vi "Core.vi"(8 "error in (no error)":errorcluster, 11 "Serial in":refnum<class "Serial.lvclass">) -> (0 "error out":errorcluster, 3 "Serial out":refnum<class "Serial.lvclass">)   [LabVIEW 2021, in "Serial.lvclass"]
uses:
  Serial.lvclass
  D:/my_projects/projects/Algorithms/Labview/21/Modbus_v121c/Network Protocol/MB/Modbus Master CR.lvclass
  MB/ctl/MB_TCP_State.ctl
  MB/Modbus Master CR.lvclass/Modbus Master CR.ctl
  MB/Status/Run/Write Run.vi
  MB/Status/write/Write write.vi
  Data Model/Device Data Model.lvclass
  MB/Modbus Master CR.lvclass
panel:
  out "MB_TCP_State":T1=enum."requests"
  in  "write enable":bool=TRUE
  in  "stop":bool
  out "stopped":bool
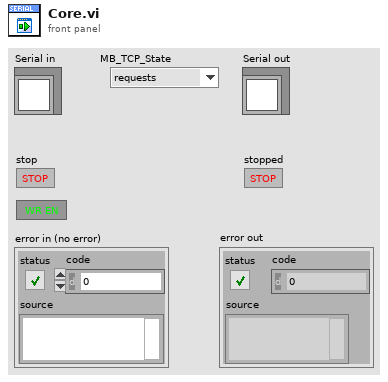
[diagram p1: front panel]
types:
  T1 = typedef "Modbus Master CR.lvclass/MB_TCP_State.ctl" = enum8{"initialization", "redefine", "standby", "ping", "connect", "wait to reconnect", "wait to reset timeout", "configure", "requests", "close connection", "stop"}
  T2 = typedef "Modbus Master CR.lvclass/MB timeouts.ctl" = cluster{"reconn_timeout":i32, "N attempt max":i32, "t_reset_TTL":i32, "period":i32}
  T3 = typedef "Modbus Master CR.lvclass/MB state.ctl" = cluster{"state":T1, "enable":bool, "Run":bool, "write enable":bool, "Write":bool, "connect":bool, "errors":i32}
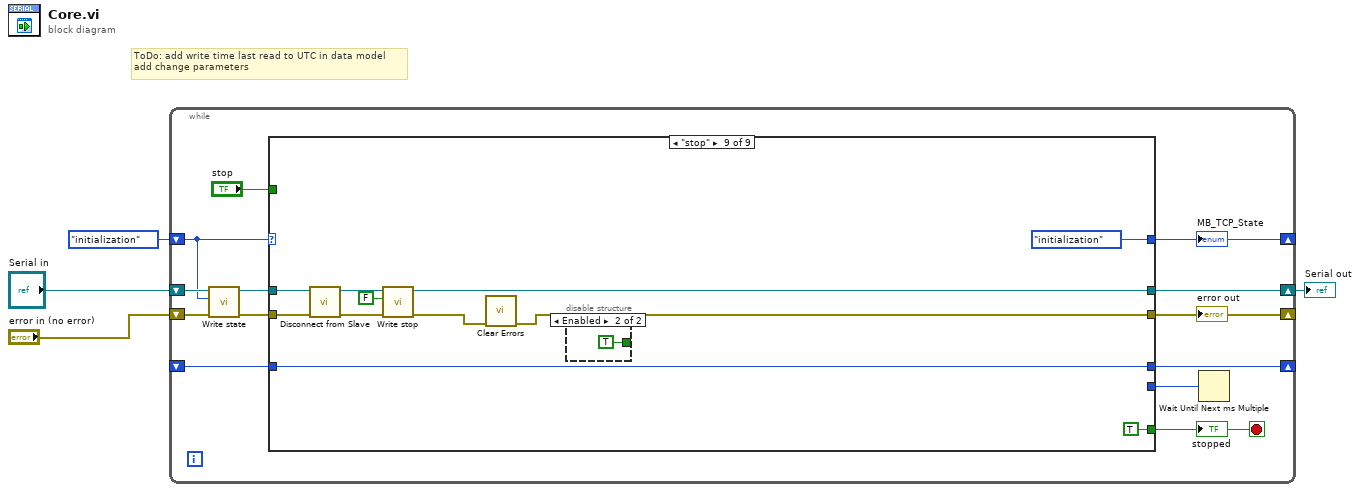
[diagram p0: block diagram]
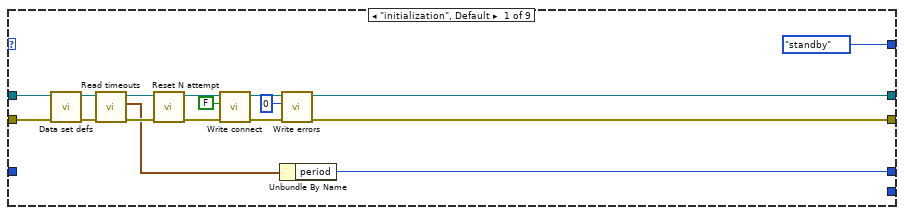
[diagram p2: hidden frame]
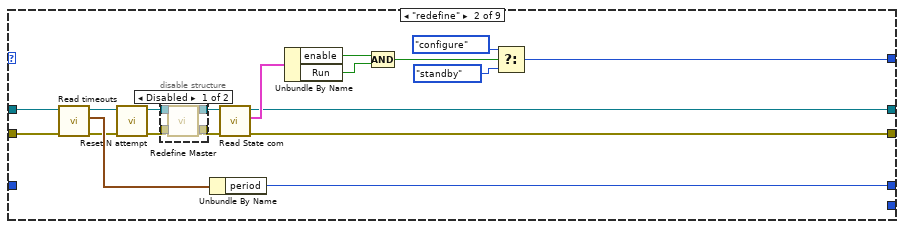
[diagram p3: hidden frame]
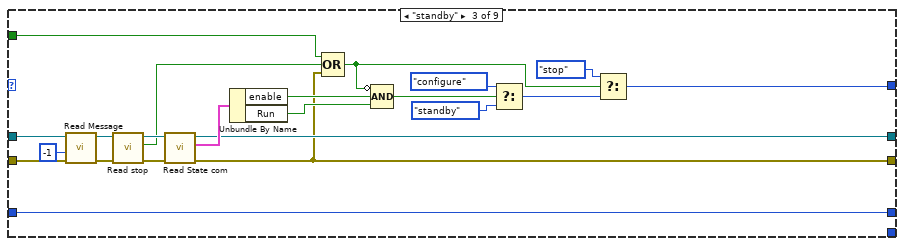
[diagram p5: hidden frame]
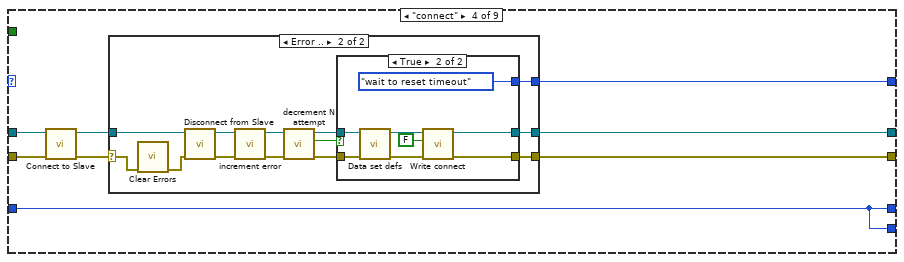
[diagram p6: hidden frame]
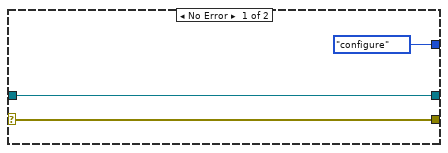
[diagram p7: hidden frame]
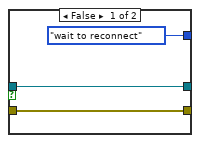
[diagram p8: hidden frame]
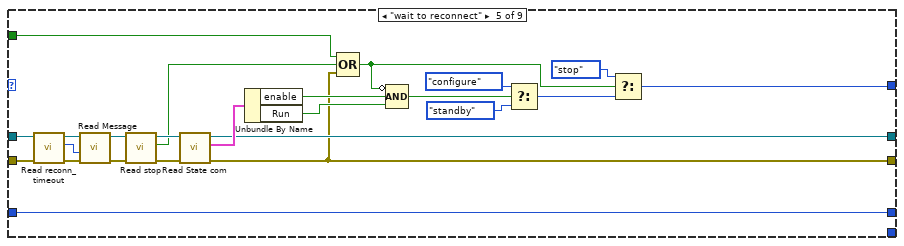
[diagram p9: hidden frame]
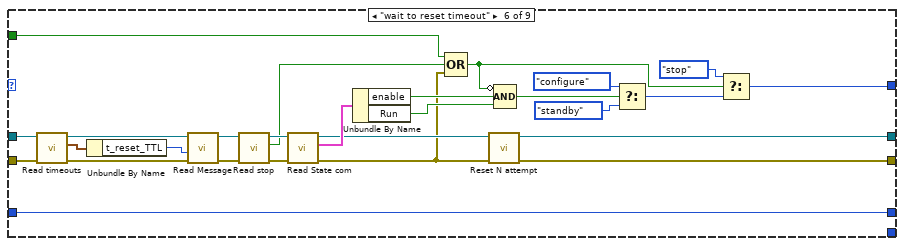
[diagram p10: hidden frame]
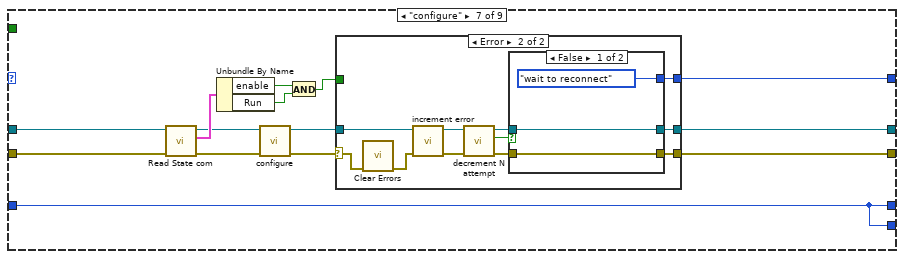
[diagram p11: hidden frame]
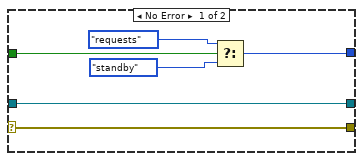
[diagram p12: hidden frame]
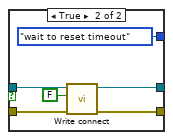
[diagram p13: hidden frame]
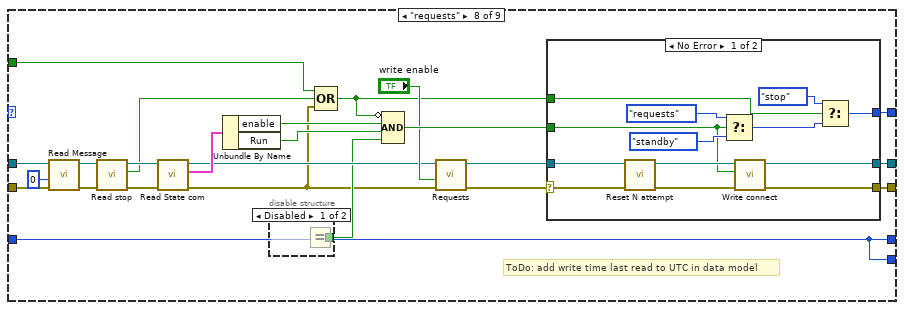
[diagram p14: hidden frame]
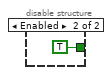
[diagram p15: hidden frame]
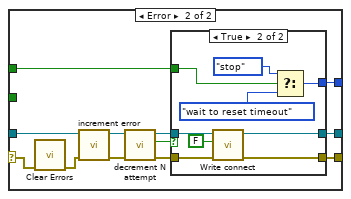
[diagram p16: hidden frame]
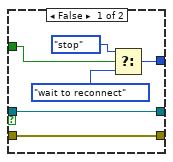
[diagram p17: hidden frame]
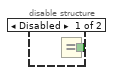
[diagram p18: hidden frame]
diagram:
  # "ToDo: add write time last read to UTC in data model\nadd change parameters"
  n1 = while {
    shift-right: [w10] -> w4
    shift-left: "Serial in" -> [w9]
    shift-right: [w11] -> _
    shift-left: "error in (no error)" -> [w7]
    shift-right: [w15] -> _
    shift-left: _ -> [w16]
    shift-right: [w12] -> _
    shift-left: MB_TCP_State."initialization" ("state") -> [w5]
    stop <- w17 stop-if-true
    n2 = call "Write state.vi"("error in (no error)"=w7, "state"=w5, "MB in"=w9) -> ("error out"=w6:errorcluster, "MB out"=w8:refnum<class "Serial.lvclass">)  [unwired: 7 in]
    n3 = case shown="\"stop\"" w5 {
      tunnel: "stop" -> [_ _ w77 _ w125 w151 _ w220 _]
      tunnel: [_ _ _ _ _ _ _ _ TRUE] -> w17
      tunnel: w8 -> [w31 w50 w67 w85 w139 w166 w174 w223 w283]
      tunnel: [w20 w36 w69 w89 w123 w143 w181 w230 w276] -> w10
      tunnel: w6 -> [w32 w49 w66 w86 w138 w165 w173 w222 w282]
      tunnel: [MB_TCP_State."standby" ("MB_TCP_State") w51 w70 w88 w124 w150 w180 w229 MB_TCP_State."initialization" ("MB_TCP_State")] -> w12
      tunnel: [w18 w37 w68 w87 w122 w142 w179 w228 w281] -> w11
      tunnel: [w33 w47 w81 w82 w140 w167 w178 w226 w284] -> w15
      tunnel: w16 -> [_ _ w81 w82 w140 w167 w178 w226 w284]
      tunnel: [_ _ _ w82 _ _ w178 w226 _] -> w14
      frame "initialization", Default {
        n4 = call "Data set defs.vi"("error in (no error)"=w32, "MB_TCP in"=w31) -> ("error out"=w26:errorcluster, "MB_TCP out"=w29:refnum<class "Serial.lvclass">)  [unwired: 8 in]
        n5 = call "Read timeouts.vi"("error in (no error)"=w26, "MB_TCP in"=w29) -> ("error out"=w30:errorcluster, "MB timeouts"=w27:T2, "MB_TCP out"=w28:refnum<class "Serial.lvclass">)  [unwired: 7 in]
        n6 = call "Reset N attempt.vi"("error in (no error)"=w30, "MB_TCP in"=w28) -> ("error out"=w24:errorcluster, "MB_TCP out"=w25:refnum<class "Serial.lvclass">)  [unwired: 8 in]
        n7 = call "Write connect.vi"("error in (no error)"=w24, "connect"=FALSE, "MB in"=w25) -> ("error out"=w22:errorcluster, "MB out"=w21:refnum<class "Serial.lvclass">)  [unwired: 7 in]
        n8 = Unbundle By Name(w27) -> ("period"=w33:i32)
        n9 = call "Write errors.vi"("error in (no error)"=w22, "errors"=0, "MB in"=w21) -> ("error out"=w18:errorcluster, "MB out"=w20:refnum<class "Serial.lvclass">)  [unwired: 7 in]
      }
      frame "redefine" {
        n10 = call "Read timeouts.vi"("error in (no error)"=w49, "MB_TCP in"=w50) -> ("error out"=w46:errorcluster, "MB timeouts"=w48:T2, "MB_TCP out"=w45:refnum<class "Serial.lvclass">)  [unwired: 7 in]
        n11 = call "Reset N attempt.vi"("error in (no error)"=w46, "MB_TCP in"=w45) -> ("error out"=w43:errorcluster, "MB_TCP out"=w44:refnum<class "Serial.lvclass">)  [unwired: 8 in]
        n12 = disable-structure shown="Disabled" {
          disable-tunnel: w44 -> [w57 w59]
          disable-tunnel: w43 -> [w56 w58]
          disable-tunnel: [w55 w59] -> w39
          disable-tunnel: [w54 w58] -> w38
          frame Disabled {
            n13 = call "Redefine Master.vi"("error in (no error)"=w56, "MB_TCP in"=w57) -> ("error out"=w54:errorcluster, "MB_TCP out"=w55:refnum<class "Serial.lvclass">)  [unwired: 8 in]
          }
          frame Enabled {
          }
        }
        n14 = Unbundle By Name(w48) -> ("period"=w47:i32)
        n15 = call "Read State com.vi"("error in (no error)"=w38, "MB_TCP in"=w39) -> ("error out"=w37:errorcluster, "State com"=w42:T3, "MB_TCP out"=w36:refnum<class "Serial.lvclass">)  [unwired: 7 in]
        n16 = Unbundle By Name(w42) -> ("enable"=w41:bool, "Run"=w40:bool)
        n17 = Compound Arithmetic op=AND(w41, w40) -> (w35:bool)
        n18 = Select(t=MB_TCP_State."configure" ("MB_TCP_State"), s=w35, f=MB_TCP_State."standby" ("MB_TCP_State")) -> (s? t:f=w51:T1)
      }
      frame "standby" {
        n19 = call "Read Message.vi"("error in (no error)"=w66, "timeout (0)"=-1, "MB in"=w67) -> ("error out"=w63:errorcluster, "MB out"=w64:refnum<class "Serial.lvclass">)  [unwired: 6 in, 1 out]
        n20 = call "Read stop.vi"("error in (no error)"=w63, "MB in"=w64) -> ("error out"=w62:errorcluster, "Stop"=w60:bool, "MB out"=w61:refnum<class "Serial.lvclass">)  [unwired: 7 in]
        n21 = call "Read State com.vi"("error in (no error)"=w62, "MB_TCP in"=w61) -> ("error out"=w68:errorcluster, "State com"=w80:T3, "MB_TCP out"=w69:refnum<class "Serial.lvclass">)  [unwired: 7 in]
        n22 = Unbundle By Name(w80) -> ("enable"=w79:bool, "Run"=w78:bool)
        n23 = Compound Arithmetic op=OR(w77, w60, w68) -> (w71:bool)
        n24 = Compound Arithmetic op=AND(invert w71, w79, w78) -> (w72:bool)
        n25 = Select(t=MB_TCP_State."configure" ("MB_TCP_State"), s=w72, f=MB_TCP_State."standby" ("MB_TCP_State")) -> (s? t:f=w73:T1)
        n26 = Select(t=MB_TCP_State."stop" ("MB_TCP_State"), s=w71, f=w73) -> (s? t:f=w70:T1)
      }
      frame "connect" {
        n27 = call-dynamic "Connect to Slave.vi"("error in (no error)"=w86, "network master in"=w85) -> ("error out"=w83:errorcluster, "network master out"=w84:refnum<class "Serial.lvclass">)  [unwired: 8 in]
        n28 = case shown="Error .." w83 {
          selector: w83 -> [w90 w97]
          tunnel: w84 -> [w91 w98]
          tunnel: [MB_TCP_State."configure" ("MB_TCP_State") w103] -> w88
          tunnel: [w91 w102] -> w89
          tunnel: [w90 w101] -> w87
          frame No Error {
          }
          frame Error {
            n29 = call <vilib>:"Clear Errors.vi"("error in (no error)"=w97) -> ("error out"=w96:errorcluster)  [unwired: 5 in, 1 out]
            n30 = call-dynamic "Disconnect from Slave.vi"("error in (no error)"=w96, "network master in"=w98) -> ("error out"=w99:errorcluster, "network master out"=w100:refnum<class "Serial.lvclass">)  [unwired: 8 in]
            n31 = call "increment error.vi"("error in (no error)"=w99, "MB_TCP in"=w100) -> ("error out"=w95:errorcluster, "MB_TCP out"=w105:refnum<class "Serial.lvclass">)  [unwired: 7 in, 1 out]
            n32 = call "decrement N attempt.vi"("error in (no error)"=w95, "MB_TCP in"=w105) -> ("error out"=w93:errorcluster, "=0"=w104:bool, "MB_TCP out"=w94:refnum<class "Serial.lvclass">)  [unwired: 7 in]
            n33 = case shown="True" w104 {
              tunnel: [MB_TCP_State."wait to reconnect" ("MB_TCP_State") MB_TCP_State."wait to reset timeout" ("MB_TCP_State")] -> w103
              tunnel: w94 -> [w107 w115]
              tunnel: [w107 w112] -> w102
              tunnel: w93 -> [w106 w114]
              tunnel: [w106 w109] -> w101
              frame False {
              }
              frame True {
                n34 = call "Data set defs.vi"("error in (no error)"=w114, "MB_TCP in"=w115) -> ("error out"=w110:errorcluster, "MB_TCP out"=w113:refnum<class "Serial.lvclass">)  [unwired: 8 in]
                n35 = call "Write connect.vi"("error in (no error)"=w110, "connect"=FALSE, "MB in"=w113) -> ("error out"=w109:errorcluster, "MB out"=w112:refnum<class "Serial.lvclass">)  [unwired: 7 in]
              }
            }
          }
        }
      }
      frame "wait to reconnect" {
        n36 = call "Read reconn_timeout.vi"("error in (no error)"=w138, "MB_TCP in"=w139) -> ("error out"=w126:errorcluster, "reconn_timeout"=w127:i32, "MB_TCP out"=w128:refnum<class "Serial.lvclass">)  [unwired: 7 in]
        n37 = call "Read Message.vi"("error in (no error)"=w126, "timeout (0)"=w127, "MB in"=w128) -> ("error out"=w120:errorcluster, "MB out"=w121:refnum<class "Serial.lvclass">)  [unwired: 6 in, 1 out]
        n38 = call "Read stop.vi"("error in (no error)"=w120, "MB in"=w121) -> ("error out"=w119:errorcluster, "Stop"=w117:bool, "MB out"=w118:refnum<class "Serial.lvclass">)  [unwired: 7 in]
        n39 = call "Read State com.vi"("error in (no error)"=w119, "MB_TCP in"=w118) -> ("error out"=w122:errorcluster, "State com"=w137:T3, "MB_TCP out"=w123:refnum<class "Serial.lvclass">)  [unwired: 7 in]
        n40 = Unbundle By Name(w137) -> ("enable"=w136:bool, "Run"=w135:bool)
        n41 = Compound Arithmetic op=OR(w125, w117, w122) -> (w129:bool)
        n42 = Compound Arithmetic op=AND(invert w129, w136, w135) -> (w130:bool)
        n43 = Select(t=MB_TCP_State."configure" ("MB_TCP_State"), s=w130, f=MB_TCP_State."standby" ("MB_TCP_State")) -> (s? t:f=w131:T1)
        n44 = Select(t=MB_TCP_State."stop" ("MB_TCP_State"), s=w129, f=w131) -> (s? t:f=w124:T1)
      }
      frame "wait to reset timeout" {
        n45 = call "Read timeouts.vi"("error in (no error)"=w165, "MB_TCP in"=w166) -> ("error out"=w154:errorcluster, "MB timeouts"=w164:T2, "MB_TCP out"=w153:refnum<class "Serial.lvclass">)  [unwired: 7 in]
        n46 = Unbundle By Name(w164) -> ("t_reset_TTL"=w152:i32)
        n47 = call "Read Message.vi"("error in (no error)"=w154, "timeout (0)"=w152, "MB in"=w153) -> ("error out"=w147:errorcluster, "MB out"=w149:refnum<class "Serial.lvclass">)  [unwired: 6 in, 1 out]
        n48 = call "Read stop.vi"("error in (no error)"=w147, "MB in"=w149) -> ("error out"=w146:errorcluster, "Stop"=w145:bool, "MB out"=w148:refnum<class "Serial.lvclass">)  [unwired: 7 in]
        n49 = call "Read State com.vi"("error in (no error)"=w146, "MB_TCP in"=w148) -> ("error out"=w141:errorcluster, "State com"=w163:T3, "MB_TCP out"=w144:refnum<class "Serial.lvclass">)  [unwired: 7 in]
        n50 = Unbundle By Name(w163) -> ("enable"=w162:bool, "Run"=w161:bool)
        n51 = Compound Arithmetic op=OR(w151, w145, w141) -> (w155:bool)
        n52 = call "Reset N attempt.vi"("error in (no error)"=w141, "MB_TCP in"=w144) -> ("error out"=w142:errorcluster, "MB_TCP out"=w143:refnum<class "Serial.lvclass">)  [unwired: 8 in]
        n53 = Compound Arithmetic op=AND(invert w155, w162, w161) -> (w156:bool)
        n54 = Select(t=MB_TCP_State."configure" ("MB_TCP_State"), s=w156, f=MB_TCP_State."standby" ("MB_TCP_State")) -> (s? t:f=w157:T1)
        n55 = Select(t=MB_TCP_State."stop" ("MB_TCP_State"), s=w155, f=w157) -> (s? t:f=w150:T1)
      }
      frame "configure" {
        n56 = call "Read State com.vi"("error in (no error)"=w173, "MB_TCP in"=w174) -> ("error out"=w171:errorcluster, "State com"=w175:T3, "MB_TCP out"=w172:refnum<class "Serial.lvclass">)  [unwired: 7 in]
        n57 = Unbundle By Name(w175) -> ("enable"=w170:bool, "Run"=w168:bool)
        n58 = call-dynamic "configure.vi"("error in (no error)"=w171, "MB_TCP in"=w172) -> ("error out"=w176:errorcluster, "MB_TCP out"=w177:refnum<class "Serial.lvclass">)  [unwired: 8 in]
        n59 = And(x=w170, y=w168) -> (x .and. y?=w169:bool)
        n60 = case shown="Error" w176 {
          selector: w176 -> [w183 w198]
          tunnel: [w187 w188] -> w180
          tunnel: [w183 w191] -> w179
          tunnel: w177 -> [w184 w190]
          tunnel: [w184 w192] -> w181
          tunnel: w169 -> [w182 _]
          frame No Error {
            n61 = Select(t=MB_TCP_State."requests" ("MB_TCP_State"), s=w182, f=MB_TCP_State."standby" ("MB_TCP_State")) -> (s? t:f=w187:T1)
          }
          frame Error {
            n62 = call <vilib>:"Clear Errors.vi"("error in (no error)"=w198) -> ("error out"=w189:errorcluster)  [unwired: 5 in, 1 out]
            n63 = call "increment error.vi"("error in (no error)"=w189, "MB_TCP in"=w190) -> ("error out"=w194:errorcluster, "MB_TCP out"=w193:refnum<class "Serial.lvclass">)  [unwired: 7 in, 1 out]
            n64 = call "decrement N attempt.vi"("error in (no error)"=w194, "MB_TCP in"=w193) -> ("error out"=w195:errorcluster, "=0"=w197:bool, "MB_TCP out"=w196:refnum<class "Serial.lvclass">)  [unwired: 7 in]
            n65 = case shown="False" w197 {
              tunnel: w196 -> [w201 w207]
              tunnel: [w201 w206] -> w192
              tunnel: w195 -> [w200 w205]
              tunnel: [w200 w203] -> w191
              tunnel: [MB_TCP_State."wait to reconnect" ("MB_TCP_State") MB_TCP_State."wait to reset timeout" ("MB_TCP_State")] -> w188
              frame False {
              }
              frame True {
                n66 = call "Write connect.vi"("error in (no error)"=w205, "connect"=FALSE, "MB in"=w207) -> ("error out"=w203:errorcluster, "MB out"=w206:refnum<class "Serial.lvclass">)  [unwired: 7 in]
              }
            }
          }
        }
      }
      frame "requests" {
        # "ToDo: add write time last read to UTC in data model"
        n67 = call "Read Message.vi"("error in (no error)"=w222, "timeout (0)"=0, "MB in"=w223) -> ("error out"=w212:errorcluster, "MB out"=w213:refnum<class "Serial.lvclass">)  [unwired: 6 in, 1 out]
        n68 = call "Read stop.vi"("error in (no error)"=w212, "MB in"=w213) -> ("error out"=w211:errorcluster, "Stop"=w209:bool, "MB out"=w210:refnum<class "Serial.lvclass">)  [unwired: 7 in]
        n69 = call "Read State com.vi"("error in (no error)"=w211, "MB_TCP in"=w210) -> ("error out"=w215:errorcluster, "State com"=w221:T3, "MB_TCP out"=w219:refnum<class "Serial.lvclass">)  [unwired: 7 in]
        n70 = Unbundle By Name(w221) -> ("enable"=w217:bool, "Run"=w216:bool)
        n71 = disable-structure shown="Disabled" {
          disable-tunnel: [w232 TRUE] -> w218
          frame Disabled {
            n72 = Equal?() -> (x = y?=w232:bool)  [unwired: 2 in]
          }
          frame Enabled {
          }
        }
        n73 = Compound Arithmetic op=OR(w220, w209, w215) -> (w208:bool)
        n74 = Compound Arithmetic op=AND(invert w208, w217, w216, w218) -> (w231:bool)
        n75 = call-dynamic "Requests.vi"("error in (no error)"=w215, "write enable"="write enable", "Serial in"=w219) -> ("error out"=w224:errorcluster, "Serial out"=w227:refnum<class "Serial.lvclass">)  [unwired: 7 in]
        n76 = case shown="No Error" w224 {
          selector: w224 -> [w243 w258]
          tunnel: [w236 w248] -> w229
          tunnel: w231 -> [w240 _]
          tunnel: [w238 w254] -> w228
          tunnel: w227 -> [w244 w251]
          tunnel: [w241 w255] -> w230
          tunnel: w208 -> [w234 w247]
          frame No Error {
            n77 = call "Reset N attempt.vi"("error in (no error)"=w243, "MB_TCP in"=w244) -> ("error out"=w239:errorcluster, "MB_TCP out"=w242:refnum<class "Serial.lvclass">)  [unwired: 8 in]
            n78 = Select(t=MB_TCP_State."requests" ("MB_TCP_State"), s=w240, f=MB_TCP_State."standby" ("MB_TCP_State")) -> (s? t:f=w235:T1)
            n79 = call "Write connect.vi"("error in (no error)"=w239, "connect"=w240, "MB in"=w242) -> ("error out"=w238:errorcluster, "MB out"=w241:refnum<class "Serial.lvclass">)  [unwired: 7 in]
            n80 = Select(t=MB_TCP_State."stop" ("MB_TCP_State"), s=w234, f=w235) -> (s? t:f=w236:T1)
          }
          frame Error {
            n81 = call <vilib>:"Clear Errors.vi"("error in (no error)"=w258) -> ("error out"=w250:errorcluster)  [unwired: 5 in, 1 out]
            n82 = call "increment error.vi"("error in (no error)"=w250, "MB_TCP in"=w251) -> ("error out"=w252:errorcluster, "MB_TCP out"=w257:refnum<class "Serial.lvclass">)  [unwired: 7 in, 1 out]
            n83 = call "decrement N attempt.vi"("error in (no error)"=w252, "MB_TCP in"=w257) -> ("error out"=w253:errorcluster, "=0"=w249:bool, "MB_TCP out"=w256:refnum<class "Serial.lvclass">)  [unwired: 7 in]
            n84 = case shown="True" w249 {
              tunnel: w256 -> [w264 w273]
              tunnel: [w264 w272] -> w255
              tunnel: w253 -> [w263 w271]
              tunnel: [w263 w269] -> w254
              tunnel: [w261 w267] -> w248
              tunnel: w247 -> [w259 w265]
              frame False {
                n85 = Select(t=MB_TCP_State."stop" ("MB_TCP_State"), s=w259, f=MB_TCP_State."wait to reconnect" ("MB_TCP_State")) -> (s? t:f=w261:T1)
              }
              frame True {
                n86 = call "Write connect.vi"("error in (no error)"=w271, "connect"=FALSE, "MB in"=w273) -> ("error out"=w269:errorcluster, "MB out"=w272:refnum<class "Serial.lvclass">)  [unwired: 7 in]
                n87 = Select(t=MB_TCP_State."stop" ("MB_TCP_State"), s=w265, f=MB_TCP_State."wait to reset timeout" ("MB_TCP_State")) -> (s? t:f=w267:T1)
              }
            }
          }
        }
      }
      frame "stop" {
        n88 = call-dynamic "Disconnect from Slave.vi"("error in (no error)"=w282, "network master in"=w283) -> ("error out"=w275:errorcluster, "network master out"=w277:refnum<class "Serial.lvclass">)  [unwired: 8 in]
        n89 = call "Write stop.vi"("error in (no error)"=w275, "Stop"=FALSE, "MB in"=w277) -> ("error out"=w274:errorcluster, "MB out"=w276:refnum<class "Serial.lvclass">)  [unwired: 7 in]
        n90 = call <vilib>:"Clear Errors.vi"("error in (no error)"=w274) -> ("error out"=w281:errorcluster)  [unwired: 5 in, 1 out]
        n91 = disable-structure shown="Enabled" {
          disable-tunnel: [w285 TRUE] -> _
          frame Disabled {
            n92 = Equal?() -> (x = y?=w285:bool)  [unwired: 2 in]
          }
          frame Enabled {
          }
        }
      }
    }
    "stopped" <- w17
    "error out" <- w11
    "MB_TCP_State" <- w12
    n93 = Wait Until Next ms Multiple(millisecond multiple=w14) -> ()  [unwired: 1 out]
  }
  "Serial out" <- w4
